vi "Voltage - Continuous Input_0209.vi"() -> ()   [LabVIEW 2021]
doc: "This example demonstrates how to continuously acquire buffered voltage measurements using a DAQmx device.\n\nFor instructions on how to connect your signals to the DAQ device, refer to your device documentation."
uses:
  <vilib>/Utility/error.llb/DialogType.ctl
  <vilib>/DAQmx/read.llb/DAQmx Read (Counter 1D DBL 1Chan NSamp).vi
  <vilib>/DAQmx/read.llb/DAQmx Read (Analog 1D Wfm NChan NSamp).vi
  <vilib>/DAQmx/create/channels.llb/DAQmx Create Channel (AI-Voltage-Basic).vi
  <vilib>/DAQmx/configure/timing.llb/DAQmx Timing (Sample Clock).vi
  <vilib>/DAQmx/miscellaneous.llb/DAQmx Fill In Error Info.vi
  <vilib>/express/express analysis/Spectral/Block/exnSpectralBlock spectral measurements power poly.vi
  <vilib>/express/express analysis/Spectral/Block/exnSpectralBlock spectral measurements power DDT.vi
  <vilib>/express/express analysis/Spectral/XNode/ExpressSpectralMeasurementsBlockNode.xnode
  <resource>/objmgr/daqmx.rc
  <vilib>/DAQmx/create/channels.llb/DAQmx Create Channel (CI-Position-Angular Encoder).vi
panel:
  in  "z index enable":bool
  out "Vib2 Spectrum":dynamicdata(graph)
  out "Vib1 Spectrum":dynamicdata(graph)
  in  "Upper Cut-Off Freq":dbl=400.0 caption="Upper Cut-Off"
  in  "Lower Cut-Off Freq":dbl=100.0 caption="Lower Cut-Off"
  out "Microphone Specrum":dynamicdata(graph)
  out "Total Spectrum":dynamicdata(graph)
  in  "Upper Cut-Off Freq":dbl=400.0 caption="Upper Cut-Off"
  in  "Lower Cut-Off Freq":dbl=100.0 caption="Lower Cut-Off"
  out "Microphone Graph":dynamicdata(graph)
  out "Encoder Data":dbl[](array[numeric])
  in  "Z Index Terminal":tag="PFI9"
  in  "B Input Terminal":tag="PFI10"
  in  "A Input Terminal":tag="PFI8"
  in  "Counter":tag="Dev1/ctr0"
  in  "Encoder Sample Clock Source":tag="PFI0"
  in  "Save Data":bool
  in  "Lower Cut-Off Freq":dbl=100.0 caption="Lower Cut-Off"
  in  "Upper Cut-Off Freq":dbl=400.0 caption="Upper Cut-Off"
  out "Time per Loop":u32
  in  "Stop":bool
  in  "Number of Samples":i32=100
  in  "Sample Rate":dbl=1000.0
  in  "AI Sample Clock Source":tag="OnboardClock"
  in  "Max Voltage":dbl=5.0
  in  "Min Voltage":dbl=-5.0
  in  "Physical Channel":tag="Dev1/ai0"
  out "Vib2":dynamicdata(graph)
  out "Vib1":dynamicdata(graph)
  # "Encoder Settings"
  # "AI Channel Settings"
  # "Filtered Vibration  Data"
  # "Filtered Vibration2  Data"
  # "Filtered Microphone  Data"
  # "Timing Settings"
  # "Microphone Spectrum"
  # "Vibration Spectrum"
  # "Vibration1 Spectrum"
  # "Vibration2 Spectrum"
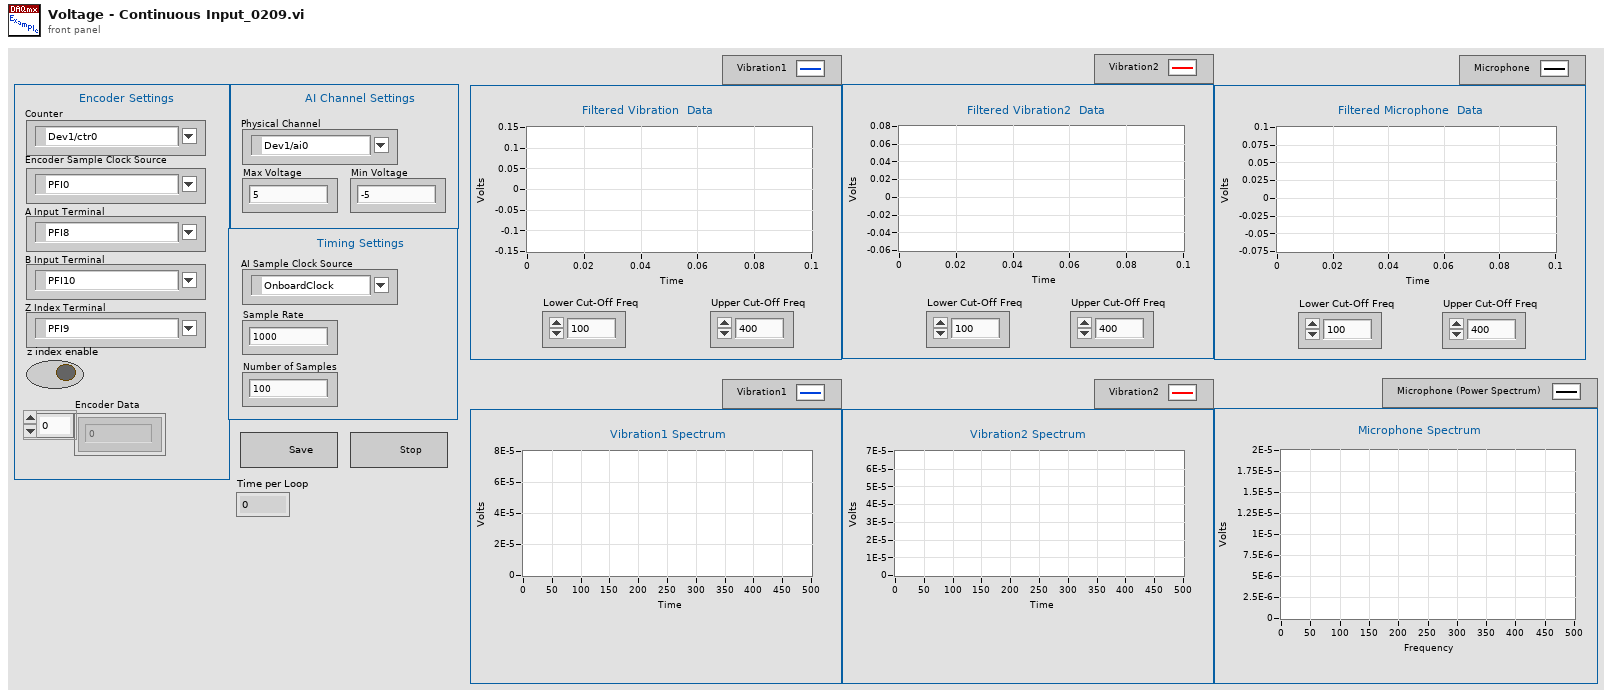
[diagram p1: front panel]
types:
  T1 = typedef "DialogType.ctl" = u16
  T2 = cluster{"averaging mode":u16, "weighting mode":u16, "number of averages":u32}
  T3 = cluster{"dB On (F)":bool, "unwrap phase (F)":bool, "convert to degree (F)":bool}
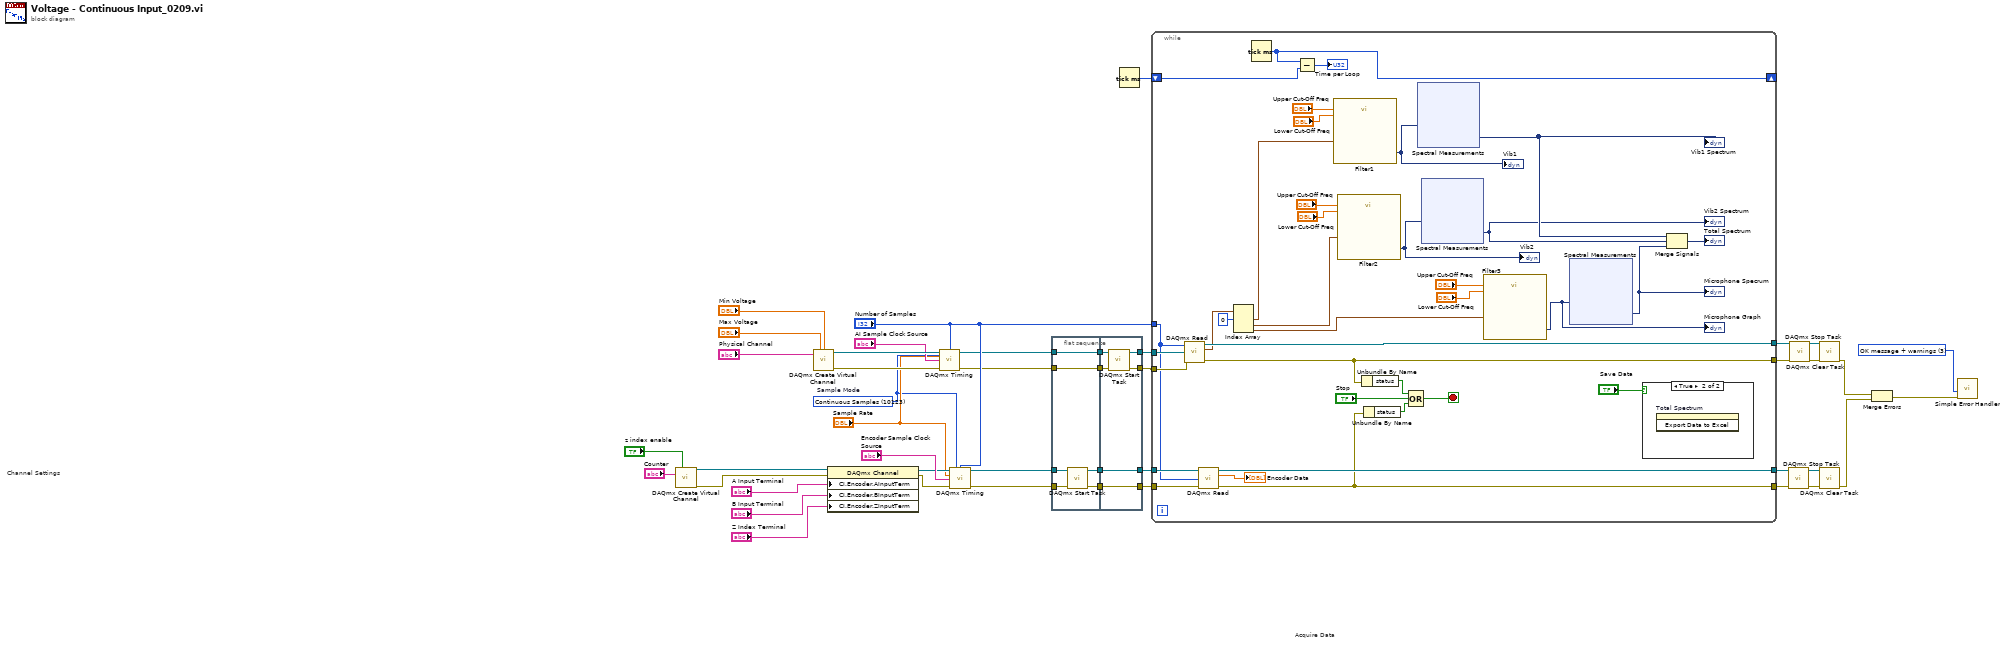
[diagram p0: block diagram]
diagram:
  w35 = T1 3 items=["no dialog", "OK message", "continue or stop message", "OK message + warnings", "continue/stop + warnings"] ("type of dialog (OK msg:1)")
  w13 = 10123 items=["Finite Samples"=10178, "Continuous Samples"=10123, "Hardware Timed Single Point"=12522]  # Sample Mode
  # "Acquire Data"
  # "Channel Settings"
  n1 = call-poly <vilib>:"DAQmx Create Virtual Channel.vi"("z index enable"="z index enable", "counter"="Counter") -> ("task out"=w30:refnum<k21>, "error out"=w28:errorcluster)  [unwired: 12 in]
  n2 = call-poly <vilib>:"DAQmx Create Virtual Channel.vi"("maximum value"="Max Voltage", "minimum value"="Min Voltage", "physical channels"="Physical Channel") -> ("task out"=w43:refnum<k21>, "error out"=w44:errorcluster)  [unwired: 11 in]
  n3 = property class="DAQmx Channel"(reference=w30, error in=w28, "CI.Encoder.AInputTerm"="A Input Terminal", "CI.Encoder.BInputTerm"="B Input Terminal", "CI.Encoder.ZInputTerm"="Z Index Terminal") -> (reference out=w25:refnum<k21>, error out=w24:errorcluster)
  n4 = call-poly <vilib>:"DAQmx Timing.vi"("task/channels in"=w43, "sample mode"=w13, "samples per channel"="Number of Samples", "rate"="Sample Rate", "source"="AI Sample Clock Source", "error in"=w44) -> ("task out"=w6:refnum<k21>, "error out"=w4:errorcluster)  [unwired: 8 in]
  n5 = call-poly <vilib>:"DAQmx Timing.vi"("task/channels in"=w25, "sample mode"=w13, "samples per channel"="Number of Samples", "rate"="Sample Rate", "source"="Encoder Sample Clock Source", "error in"=w24) -> ("task out"=w3:refnum<k21>, "error out"=w2:errorcluster)  [unwired: 8 in]
  n6 = flat-sequence {
    tunnel: [w50] -> w11
    tunnel: [w49] -> w10
    tunnel: [w48] -> w7
    tunnel: w6 -> [w48]
    tunnel: w4 -> [w47]
    tunnel: [w47] -> w5
    tunnel: w3 -> [w46]
    tunnel: w2 -> [w45]
    tunnel: [w55] -> w20
    tunnel: [w56] -> w21
    tunnel: w11 -> [w56]
    tunnel: w10 -> [w55]
    tunnel: [w54] -> w9
    tunnel: [w53] -> w8
    tunnel: w7 -> [w52]
    tunnel: w5 -> [w51]
    frame #0 {
      n7 = call <vilib>:"DAQmx Start Task.vi"("task/channels in"=w46, "error in"=w45) -> ("task out"=w50:refnum<k21>, "error out"=w49:errorcluster)  [unwired: 12 in]
    }
    frame #1 {
      n8 = call <vilib>:"DAQmx Start Task.vi"("task/channels in"=w52, "error in"=w51) -> ("task out"=w54:refnum<k21>, "error out"=w53:errorcluster)  [unwired: 12 in]
    }
  }
  n9 = Tick Count (ms)() -> (millisecond timer value=w34:u32)
  n10 = while {
    tunnel: w9 -> [w92]
    tunnel: w8 -> [w91]
    tunnel: [w90] -> w38
    tunnel: [w89] -> w33
    tunnel: "Number of Samples" -> [w74]
    shift-right: [w87] -> _
    shift-left: w34 -> [w88]
    tunnel: w21 -> [w82]
    tunnel: w20 -> [w81]
    tunnel: [w80] -> w19
    tunnel: [w79] -> w18
    stop <- w75 stop-if-true
    n11 = call-poly <vilib>:"DAQmx Read.vi"("task/channels in"=w92, "number of samples per channel"=w74, "error in"=w91) -> ("task out"=w90:refnum<k21>, "data"=w73:waveform(dbl)[], "error out"=w89:errorcluster)  [unwired: 10 in]
    n12 = call-poly <vilib>:"DAQmx Read.vi"("task/channels in"=w82, "number of samples per channel"=w74, "error in"=w81) -> ("task out"=w80:refnum<k21>, "data"=→"Encoder Data":dbl[], "error out"=w79:errorcluster)  [unwired: 10 in]
    n13 = Index Array(array=w73, index #1=0 ("index")) -> (element #1=w61:waveform(dbl), element #2=w64:waveform(dbl), element #3=w71:waveform(dbl))  [unwired: 2 in]
    n14 = Tick Count (ms)() -> (millisecond timer value=w87:u32)
    n15 = Subtract(x=w87, y=w88) -> (x-y=→"Time per Loop":u32)
    n16 = call "Filter1"("Lower Cut-Off"="Lower Cut-Off Freq", "Upper Cut-Off"="Upper Cut-Off Freq", "Signal"=w61) -> ("Filtered Signal"=w60:dynamicdata)  [unwired: 7 in, 1 out]
    "Vib1" <- w60
    n17 = call "Filter2"("Lower Cut-Off"="Lower Cut-Off Freq", "Upper Cut-Off"="Upper Cut-Off Freq", "Signal"=w64) -> ("Filtered Signal"=w59:dynamicdata)  [unwired: 7 in, 1 out]
    "Vib2" <- w59
    n18 = Unbundle By Name(w89) -> ("status"=w78:bool)
    n19 = Unbundle By Name(w79) -> ("status"=w76:bool)
    n20 = Compound Arithmetic op=OR(w78, "Stop", w76) -> (w75:bool)
    n21 = xnode "Spectral Measurements"("Signals"=w60) -> ("Power Spectrum"=w58:dynamicdata)  [unwired: 1 in, 1 out]
    "Vib1 Spectrum" <- w58
    n22 = xnode "Spectral Measurements"("Signals"=w59) -> ("Power Spectrum"=w57:dynamicdata)  [unwired: 1 in, 1 out]
    "Vib2 Spectrum" <- w57
    n23 = call "Filter3"("Lower Cut-Off"="Lower Cut-Off Freq", "Upper Cut-Off"="Upper Cut-Off Freq", "Signal"=w71) -> ("Filtered Signal"=w68:dynamicdata)  [unwired: 7 in, 1 out]
    "Microphone Graph" <- w68
    n24 = xnode "Spectral Measurements"("Signals"=w68) -> ("Power Spectrum"=w65:dynamicdata)  [unwired: 1 in, 1 out]
    "Microphone Specrum" <- w65
    n25 = case shown="True" "Save Data" {
      frame False {
      }
      frame True {
        n26 = invoke on="Total Spectrum" class="WFGraph (strict)" method="Export Data to Excel"() -> ()  [unwired: 3 in, 3 out]
      }
    }
    n27 = Merge Signals(w58, w57, w65) -> (→"Total Spectrum":dynamicdata)
  }
  n28 = call <vilib>:"DAQmx Stop Task.vi"("task/channels in"=w19, "error in"=w18) -> ("task out"=w22:refnum<k21>, "error out"=w23:errorcluster)  [unwired: 12 in]
  n29 = call <vilib>:"DAQmx Stop Task.vi"("task/channels in"=w38, "error in"=w33) -> ("task out"=w36:refnum<k21>, "error out"=w37:errorcluster)  [unwired: 12 in]
  n30 = call <vilib>:"DAQmx Clear Task.vi"("task in"=w36, "error in"=w37) -> ("error out"=w17:errorcluster)  [unwired: 13 in]
  n31 = call <vilib>:"DAQmx Clear Task.vi"("task in"=w22, "error in"=w23) -> ("error out"=w16:errorcluster)  [unwired: 13 in]
  n32 = Merge Errors(w17, w16) -> (w15:errorcluster)
  n33 = call <vilib>:"Simple Error Handler.vi"("type of dialog (OK msg:1)"=w35, "error in (no error)"=w15) -> ()  [unwired: 3 in, 5 out]
